vi "fake tool broken vi.vi"   [LabVIEW 2020, in "MCP Server tests.lvlib"]
doc: "This is a fake tool to test the MCP server toolkit. It's a broken VI by purpouse to test resiliance of the server against this."
uses:
  MCP Server tests.lvlib
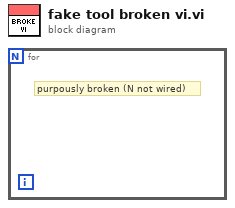
[diagram p0: block diagram]
diagram:
  n1 = for {
    # "purpously broken (N not wired)"
  }
